vi "parse_cmd_from_file.vi"(8 "error in (no error)":errorcluster, 10 "Command List Filepath":path=path "D:/Program Files (x86)/National Instruments/LabVIEW 2011/instr.lib/Agilent MXA Series/express/CommandList.xml") -> (0 "Group":string[](array[string]), 1 "Property":string[](array[string]), 2 "Result Command Array":T1)   [LabVIEW 2018]
uses:
  command_spec.ctl
  <vilib>/xml/Load XML File.vi
  <vilib>/xml/Close Reference(Node).vi
  <vilib>/xml/NI_XML.lvlib
  <resource>/objmgr/DOMUserDefRef.rc
panel:
  out "SCPI Command":string[](array[string])
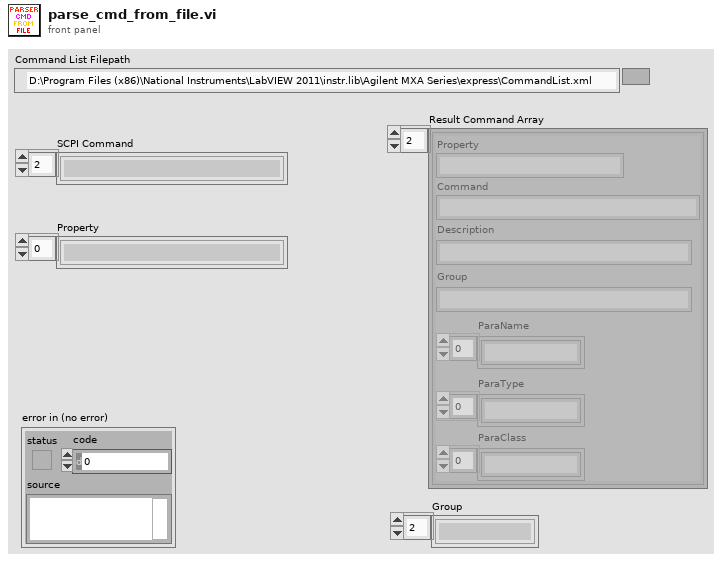
[diagram p1: front panel]
types:
  T1 = typedef "command_spec.ctl" = cluster{"Property":string, "Command":string, "Description":string, "Group":string, "ParaName":string[], "ParaType":string[], "ParaClass":string[]}[]
  T2 = cluster{"Property":string, "SCPI Command":string, "Description":string, "Group":string, "ParaName":string[], "ParaType":string[], "ParaClass":string[]}
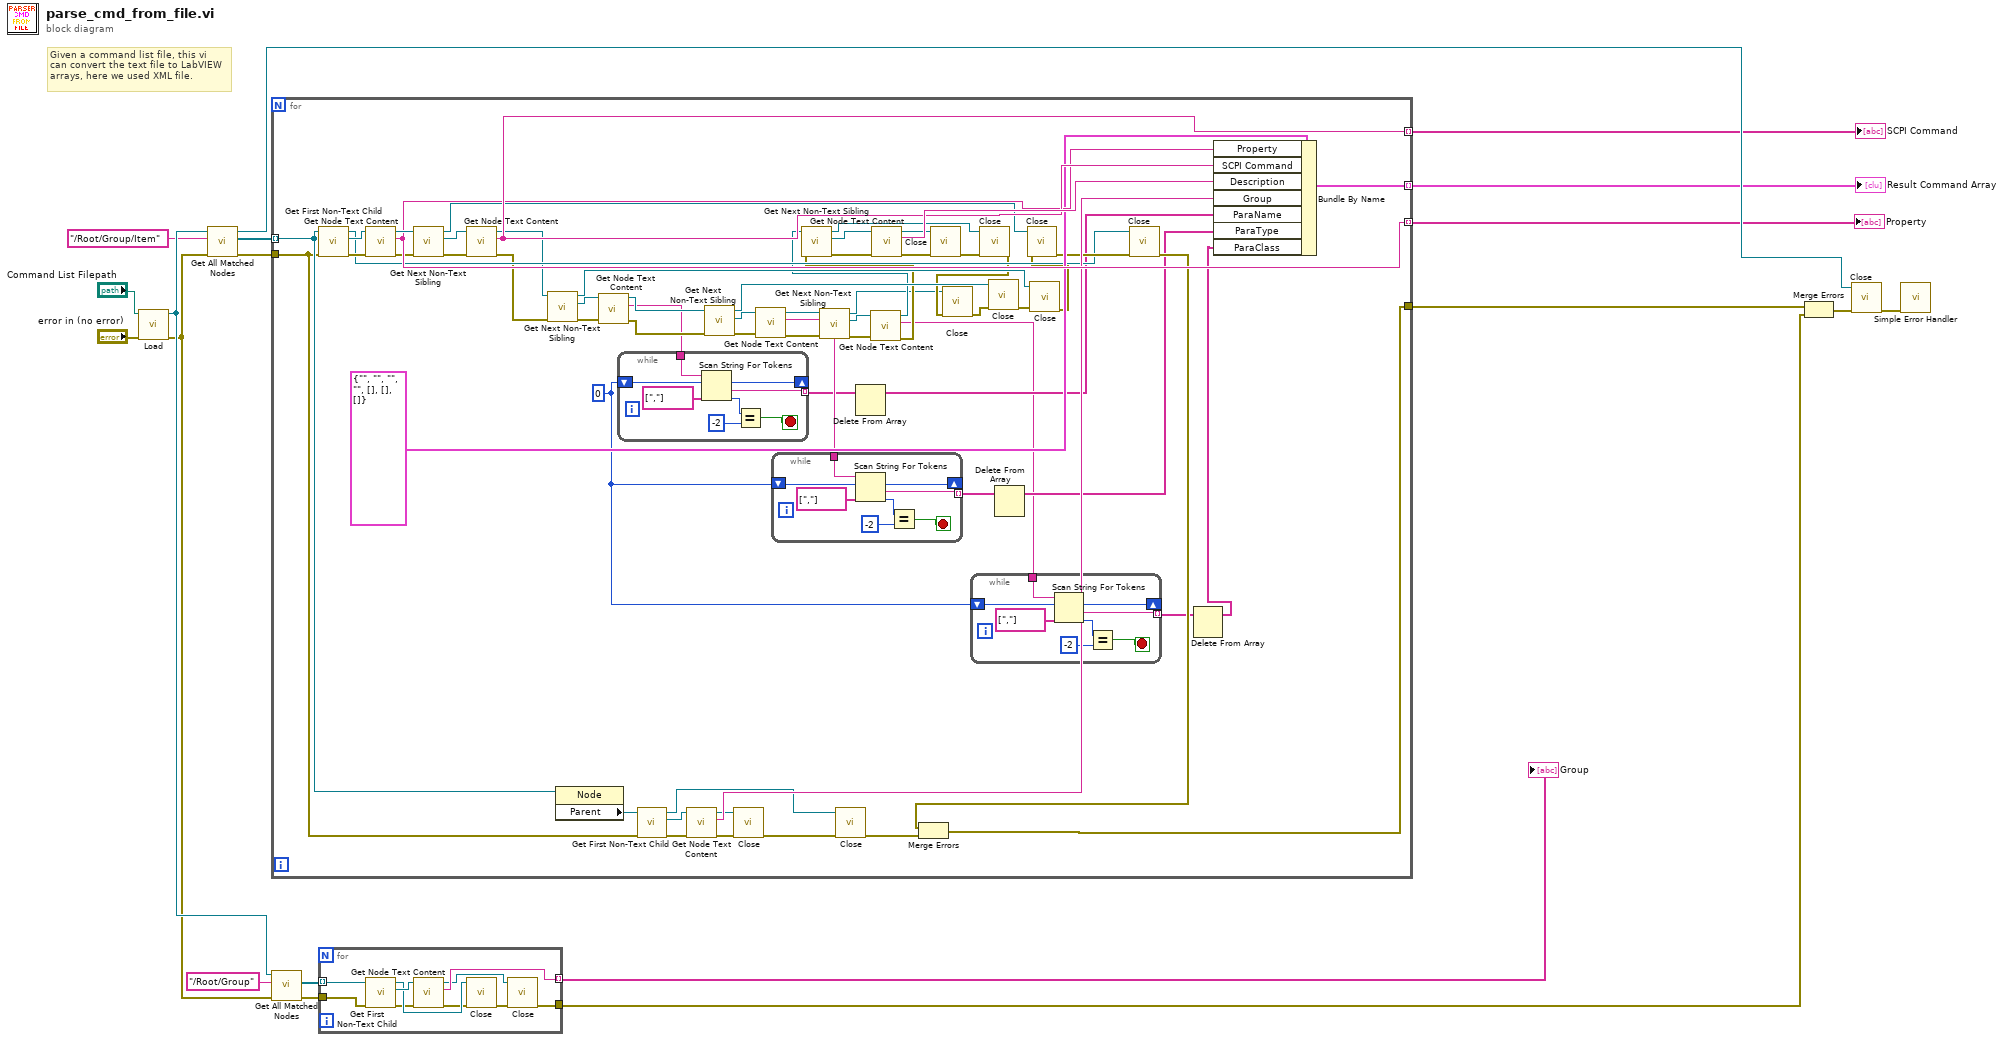
[diagram p0: block diagram]
diagram:
  # "Given a command list file, this vi\ncan convert the text file to LabVIEW\narrays, here we used XML file."
  n1 = call-poly <vilib>:"Load.vi"("path to XML document"="Command List Filepath", "error in (no error)"="error in (no error)") -> ("DOM document out"=w11:refnum<k20>, "error out"=w9:errorcluster)  [unwired: 11 in, 1 out]
  n2 = call <vilib>:"Get All Matched Nodes.vi"("error in (no error)"=w9, "XPath expression"="/Root/Group/Item", "node in"=w11) -> ("error out"=w16:errorcluster, "node result array"=w17:refnum<k20>[], "node out"=w18:refnum<k20>)  [unwired: 6 in]
  n3 = for {
    tunnel: w17 -> [w70] mode=indexing
    tunnel: w16 -> [w59]
    tunnel: [w76] -> w14 mode=indexing
    tunnel: [w77] -> w13 mode=indexing
    tunnel: [w74] -> w1 mode=indexing
    tunnel: [w51] -> w3
    w20 = 0 ("offset past token")
    n4 = call <vilib>:"Get First Non-Text Child.vi"("error in (no error)"=w59, "node in"=w70) -> ("error out"=w82:errorcluster, "child node"=w83:refnum<k20>, "node out"=w60:refnum<k20>)  [unwired: 6 in, 1 out]
    n5 = call <vilib>:"Get Node Text Content.vi"("error in (no error)"=w82, "node in"=w83) -> ("error out"=w73:errorcluster, "node text"=w76:string, "node out"=w81:refnum<k20>)  [unwired: 7 in]
    n6 = call <vilib>:"Get Next Non-Text Sibling.vi"("error in (no error)"=w73, "node in"=w81) -> ("error out"=w72:errorcluster, "sibling node"=w80:refnum<k20>, "node out"=w62:refnum<k20>)  [unwired: 6 in, 1 out]
    n7 = call <vilib>:"Get Node Text Content.vi"("error in (no error)"=w72, "node in"=w80) -> ("error out"=w49:errorcluster, "node text"=w77:string, "node out"=w50:refnum<k20>)  [unwired: 7 in]
    n8 = call <vilib>:"Get Next Non-Text Sibling.vi"("error in (no error)"=w49, "node in"=w50) -> ("error out"=w47:errorcluster, "sibling node"=w48:refnum<k20>, "node out"=w38:refnum<k20>)  [unwired: 6 in, 1 out]
    n9 = property class="Node"(reference=w70) -> ("Parent"=w69:refnum<k20>)  [unwired: 1 in, 2 out]
    n10 = call <vilib>:"Get Node Text Content.vi"("error in (no error)"=w47, "node in"=w48) -> ("error out"=w43:errorcluster, "node text"=w42:string, "node out"=w44:refnum<k20>)  [unwired: 7 in]
    n11 = while {
      tunnel: [w107] -> w36 mode=indexing
      shift-right: [w103] -> _
      shift-left: w20 -> [w106]
      tunnel: w42 -> [w101]
      stop <- w104 stop-if-true
      n12 = Scan String For Tokens(6:string[] [","] ("delimiters (\\s,\\t,\\r,\\n)"), 8:w106, 9:w101) -> (0:w102:i32, 1:w107:string, 2:w103:i32)  [unwired: 3 in, 1 out]
      n13 = Equal?(x=w102, y=-2) -> (x = y?=w104:bool)
    }
    n14 = call <vilib>:"Get First Non-Text Child.vi"("error in (no error)"=w59, "node in"=w69) -> ("error out"=w58:errorcluster, "child node"=w68:refnum<k20>, "node out"=w54:refnum<k20>)  [unwired: 6 in, 1 out]
    n15 = call <vilib>:"Get Node Text Content.vi"("error in (no error)"=w58, "node in"=w68) -> ("error out"=w56:errorcluster, "node text"=w67:string, "node out"=w57:refnum<k20>)  [unwired: 7 in]
    n16 = call <vilib>:"Get Next Non-Text Sibling.vi"("error in (no error)"=w43, "node in"=w44) -> ("error out"=w45:errorcluster, "sibling node"=w46:refnum<k20>, "node out"=w40:refnum<k20>)  [unwired: 6 in, 1 out]
    n17 = call-poly <vilib>:"Close.vi"("error in (no error)"=w56, "node"=w57) -> ("error out"=w55:errorcluster)  [unwired: 7 in]
    n18 = call <vilib>:"Get Node Text Content.vi"("error in (no error)"=w45, "node in"=w46) -> ("error out"=w28:errorcluster, "node text"=w41:string, "node out"=w29:refnum<k20>)  [unwired: 7 in]
    n19 = while {
      tunnel: [w99] -> w34 mode=indexing
      shift-right: [w95] -> _
      shift-left: w20 -> [w98]
      tunnel: w41 -> [w93]
      stop <- w96 stop-if-true
      n20 = Scan String For Tokens(6:string[] [","] ("delimiters (\\s,\\t,\\r,\\n)"), 8:w98, 9:w93) -> (0:w94:i32, 1:w99:string, 2:w95:i32)  [unwired: 3 in, 1 out]
      n21 = Equal?(x=w94, y=-2) -> (x = y?=w96:bool)
    }
    n22 = call <vilib>:"Get Next Non-Text Sibling.vi"("error in (no error)"=w28, "node in"=w29) -> ("error out"=w30:errorcluster, "sibling node"=w31:refnum<k20>, "node out"=w21:refnum<k20>)  [unwired: 6 in, 1 out]
    n23 = call-poly <vilib>:"Close.vi"("error in (no error)"=w55, "node"=w54) -> ("error out"=w53:errorcluster)  [unwired: 7 in]
    n24 = Delete From Array(array=w36) -> (array with subset deleted=w35:string[])  [unwired: 2 in, 1 out]
    n25 = call <vilib>:"Get Node Text Content.vi"("error in (no error)"=w30, "node in"=w31) -> ("error out"=w26:errorcluster, "node text"=w25:string, "node out"=w27:refnum<k20>)  [unwired: 7 in]
    n26 = call <vilib>:"Get Next Non-Text Sibling.vi"("error in (no error)"=w26, "node in"=w27) -> ("error out"=w71:errorcluster, "sibling node"=w79:refnum<k20>, "node out"=w64:refnum<k20>)  [unwired: 6 in, 1 out]
    n27 = call <vilib>:"Get Node Text Content.vi"("error in (no error)"=w71, "node in"=w79) -> ("error out"=w65:errorcluster, "node text"=w78:string, "node out"=w66:refnum<k20>)  [unwired: 7 in]
    n28 = call-poly <vilib>:"Close.vi"("error in (no error)"=w65, "node"=w66) -> ("error out"=w63:errorcluster)  [unwired: 7 in]
    n29 = while {
      tunnel: [w91] -> w32 mode=indexing
      shift-right: [w87] -> _
      shift-left: w20 -> [w90]
      tunnel: w25 -> [w85]
      stop <- w88 stop-if-true
      n30 = Scan String For Tokens(6:string[] [","] ("delimiters (\\s,\\t,\\r,\\n)"), 8:w90, 9:w85) -> (0:w86:i32, 1:w91:string, 2:w87:i32)  [unwired: 3 in, 1 out]
      n31 = Equal?(x=w86, y=-2) -> (x = y?=w88:bool)
    }
    n32 = call-poly <vilib>:"Close.vi"("error in (no error)"=w63, "node"=w64) -> ("error out"=w22:errorcluster)  [unwired: 7 in]
    n33 = call-poly <vilib>:"Close.vi"("error in (no error)"=w22, "node"=w21) -> ("error out"=w23:errorcluster)  [unwired: 7 in]
    n34 = call-poly <vilib>:"Close.vi"("error in (no error)"=w23, "node"=w40) -> ("error out"=w39:errorcluster)  [unwired: 7 in]
    n35 = Delete From Array(array=w34) -> (array with subset deleted=w33:string[])  [unwired: 2 in, 1 out]
    n36 = call-poly <vilib>:"Close.vi"("error in (no error)"=w39, "node"=w38) -> ("error out"=w37:errorcluster)  [unwired: 7 in]
    n37 = call-poly <vilib>:"Close.vi"("error in (no error)"=w37, "node"=w62) -> ("error out"=w61:errorcluster)  [unwired: 7 in]
    n38 = call-poly <vilib>:"Close.vi"("error in (no error)"=w61, "node"=w60) -> ("error out"=w52:errorcluster)  [unwired: 7 in]
    n39 = Merge Errors(w52, w53) -> (w51:errorcluster)
    n40 = Delete From Array(array=w32) -> (array with subset deleted=w24:string[])  [unwired: 2 in, 1 out]
    n41 = Bundle By Name(cluster=T2 {"Property"="", "SCPI Command"="", "Description"="", "Group"="", "ParaName"=[], "ParaType"=[], "ParaClass"=[]} ("Cluster"), "Property"=w76, "SCPI Command"=w77, "Description"=w78, "Group"=w67, "ParaName"=w35, "ParaType"=w33, "ParaClass"=w24) -> (w74:T2)
  }
  "Result Command Array" <- w1
  "Property" <- w14
  "SCPI Command" <- w13
  n42 = call <vilib>:"Get All Matched Nodes.vi"("error in (no error)"=w9, "XPath expression"="/Root/Group", "node in"=w11) -> ("error out"=w5:errorcluster, "node result array"=w7:refnum<k20>[])  [unwired: 6 in, 1 out]
  n43 = for {
    tunnel: w7 -> [w117] mode=indexing
    tunnel: [w115] -> w6 mode=indexing
    tunnel: [w109] -> w4
    tunnel: w5 -> [w108]
    n44 = call <vilib>:"Get First Non-Text Child.vi"("error in (no error)"=w108, "node in"=w117) -> ("error out"=w112:errorcluster, "child node"=w116:refnum<k20>, "node out"=w114:refnum<k20>)  [unwired: 6 in, 1 out]
    n45 = call <vilib>:"Get Node Text Content.vi"("error in (no error)"=w112, "node in"=w116) -> ("error out"=w111:errorcluster, "node text"=w115:string, "node out"=w113:refnum<k20>)  [unwired: 7 in]
    n46 = call-poly <vilib>:"Close.vi"("error in (no error)"=w111, "node"=w114) -> ("error out"=w110:errorcluster)  [unwired: 7 in]
    n47 = call-poly <vilib>:"Close.vi"("error in (no error)"=w110, "node"=w113) -> ("error out"=w109:errorcluster)  [unwired: 7 in]
  }
  "Group" <- w6
  n48 = Merge Errors(w3, w4) -> (w2:errorcluster)
  n49 = call-poly <vilib>:"Close.vi"("error in (no error)"=w2, "node"=w18) -> ("error out"=w15:errorcluster)  [unwired: 7 in]
  n50 = call <vilib>:"Simple Error Handler.vi"("error in (no error)"=w15) -> ()  [unwired: 4 in, 5 out]
